vi "initShootFromGlobalVariables.vi"(9 "Numeric":u32, 10 "Shooting":bool, 11 "Shoot":bool) -> (2 "f":u32, 3 "Boolean":bool)   [LabVIEW 2014]
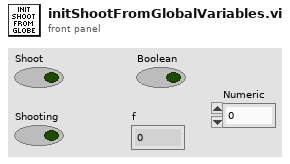
[diagram p1: front panel]
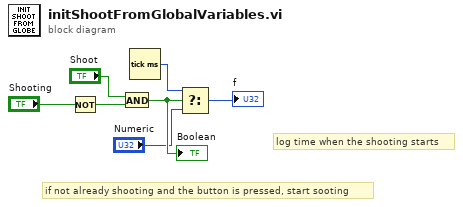
[diagram p0: block diagram]
diagram:
  # "log time when the shooting starts"
  # "if not already shooting and the button is pressed, start sooting"
  n1 = Not(x="Shooting") -> (.not. x?=w6:bool)
  n2 = And(x="Shoot", y=w6) -> (x .and. y?=w4:bool)
  "Boolean" <- w4
  n3 = Tick Count (ms)() -> (millisecond timer value=w2:u32)
  n4 = Select(t=w2, s=w4, f="Numeric") -> (s? t:f=→"f":u32)
